vi "Get Library Items.vi"(7 "Calling VI Ref":refnum<vi>, 8 "error in (no error)":errorcluster, 11 "Path":path) -> (0 "error out":errorcluster, 2 "Cancelled?":bool, 3 "Items Data":refnum<class "Item.lvclass">[](array[class]))   [LabVIEW 2020, in "VI Properties Editor.lvlib"]
doc: "Initializes class data for all items contained within the library or class identified by <B>Path</B>."
uses:
  VI Properties Editor.lvlib
  Classes/Item/Item.lvclass
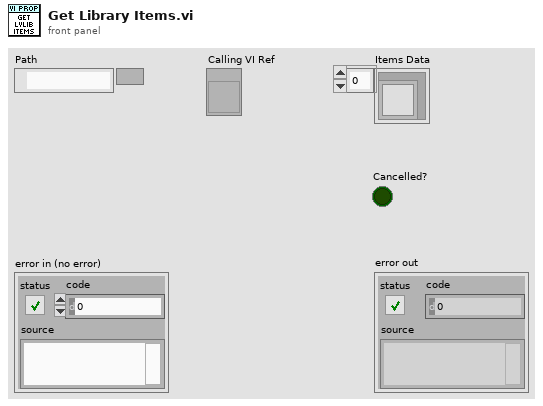
[diagram p1: front panel]
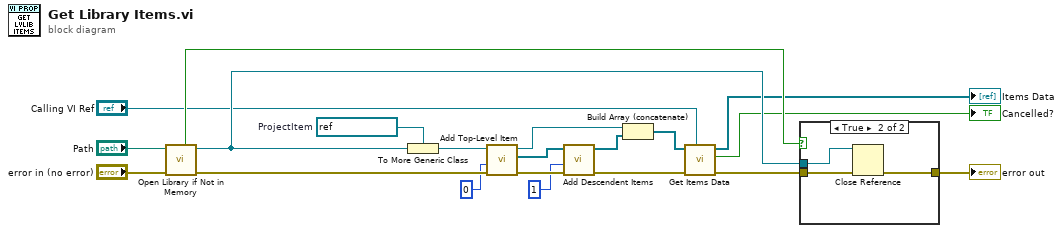
[diagram p0: block diagram]
diagram:
  w12 = refnum<vi> refnum  # ProjectItem
  n1 = call "Open Library if Not in Memory.vi"("error in (no error)"="error in (no error)", "Path"="Path") -> ("error out"=w10:errorcluster, "Library Ref"=w20:refnum<vi>, "Opened?"=w15:bool)  [unwired: 7 in]
  n2 = To More Generic Class(target class=w12, reference=w20) -> (generic class reference=w9:refnum<vi>)
  n3 = call "Add Top-Level Item.vi"("error in (no error)"=w10, "Order"=0, "ProjectItem Ref"=w9) -> ("error out"=w19:errorcluster, "Descendents Refs"=w4:refnum<vi>[], "Item"=w7:refnum<class "Item.lvclass">)  [unwired: 6 in]
  n4 = call "Add Descendent Items.vi"("error in (no error)"=w19, "Order"=1, "Descendents Refs"=w4) -> ("error out"=w2:errorcluster, "Items"=w6:refnum<class "Item.lvclass">[])  [unwired: 7 in]
  n5 = Build Array (concatenate)(w7, w6) -> (w5:refnum<class "Item.lvclass">[])
  n6 = call "Get Items Data.vi"("Calling VI Ref"="Calling VI Ref", "error in (no error)"=w2, "Items"=w5) -> ("error out"=w14:errorcluster, "Cancelled?"=→"Cancelled?":bool, "Items out"=→"Items Data":refnum<class "Item.lvclass">[])  [unwired: 6 in]
  n7 = case shown="True" w15 {
    tunnel: w14 -> [w21 w24]
    tunnel: w20 -> [_ w23]
    tunnel: [w21 w22] -> w16
    frame False {
    }
    frame True {
      n8 = Close Reference(reference=w23, error in (no error)=w24) -> (error out=w22:errorcluster)
    }
  }
  "error out" <- w16
